vi "FPGA_AIWriteAccumulatorReset.vi"(8 "error in (no error)":errorcluster, 10 "Channel":T1, 11 "AI Reference in":T2) -> (0 "error out":errorcluster, 3 "AI Reference out":T2)   [LabVIEW 2017]
uses:
  <vilib>/Rock Robotics/SystemInterfaces/AI/FPGA_AIDevRef.ctl
  <vilib>/Rock Robotics/SystemInterfaces/AI/FPGA_AIChannel.ctl
  <vilib>/Rock Robotics/SystemInterfaces/System/FPGA_SystemFPGA Ref Global.vi
  <vilib>/Utility/error.llb/Error Cluster From Error Code.vi
  <vilib>/rvi/errors/niLvFpgaAdjustHostInterfaceError.vi
  <vilib>/rvi/interface/nirviReadWriteControl/nirviReadWriteControl.xnode
  <vilib>/Rock Robotics/SystemInterfaces/System/FPGA_SystemFRC FPGA Ref.ctl
  <vilib>/rvi/interface/Simulation/niFpgaSimulationCallBeginRW.vi
  NiFpgaLv.dll
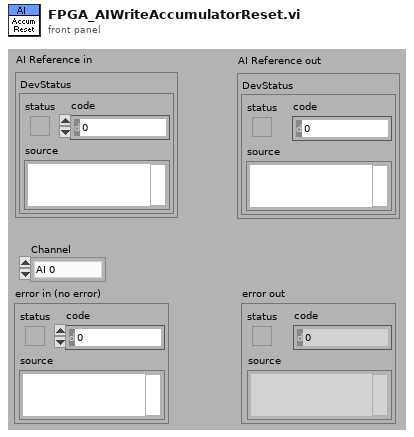
[diagram p1: front panel]
types:
  T1 = typedef "FPGA_AIChannel.ctl" = enum8{"AI 0", "AI 1", "AI 2", "AI 3", "AI MXP 0", "AI MXP 1", "AI MXP 2", "AI MXP 3", "Invalid"}
  T2 = typedef "FPGA_AIDevRef.ctl" = cluster{"DevStatus":errorcluster}
  T3 = typedef "FPGA_SystemFRC FPGA Ref.ctl" = refnum<k20>
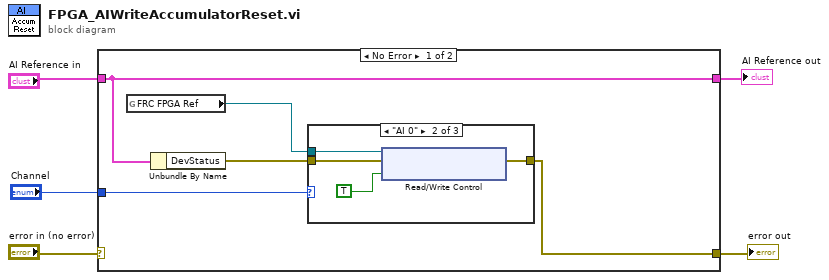
[diagram p0: block diagram]
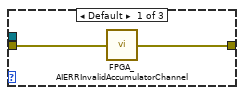
[diagram p2: hidden frame]
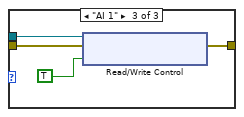
[diagram p3: hidden frame]
diagram:
  n1 = case shown="No Error" "error in (no error)" {
    selector: "error in (no error)" -> [_ w21]
    tunnel: [w10 w22] -> w4
    tunnel: "AI Reference in" -> [w10 w22]
    tunnel: [w8 w21] -> w2
    tunnel: "Channel" -> [w7 _]
    frame No Error {
      n2 = global read "FPGA_SystemFPGA Ref Global.vi" "FRC FPGA Ref"() -> (w6:T3)
      n3 = Unbundle By Name(w10) -> ("DevStatus"=w9:errorcluster)
      n4 = case shown="\"AI 0\"" w7 {
        tunnel: w9 -> [w12 w14 w18]
        tunnel: [w11 w16 w20] -> w8
        tunnel: w6 -> [_ w13 w17]
        frame Default {
          n5 = call <vilib>:"FPGA_AIERRInvalidAccumulatorChannel.vi"("error in (no error)"=w12) -> ("error out"=w11:errorcluster)
        }
        frame "AI 0" {
          n6 = xnode "Read/Write Control"("FPGA VI Reference In"=w13, "error in"=w14, "Accumulator0.Reset"=TRUE) -> ("error out"=w16:errorcluster)  [unwired: 1 out]
        }
        frame "AI 1" {
          n7 = xnode "Read/Write Control"("FPGA VI Reference In"=w17, "error in"=w18, "Accumulator1.Reset"=TRUE) -> ("error out"=w20:errorcluster)  [unwired: 1 out]
        }
      }
    }
    frame Error {
    }
  }
  "AI Reference out" <- w4
  "error out" <- w2
